vi "ook.vi"() -> ()   [LabVIEW 2009]
panel:
  out "合成波":cluster{dbl[], dbl[]}(graph)
  out "XYグラフ 3":cluster{dbl[], dbl[]}(graph) caption="XYグラフ"
  out "XYグラフ 2":cluster{dbl[], dbl[]}(graph) caption="XYグラフ"
  out "XYグラフ":cluster{dbl[], dbl[]}(graph)
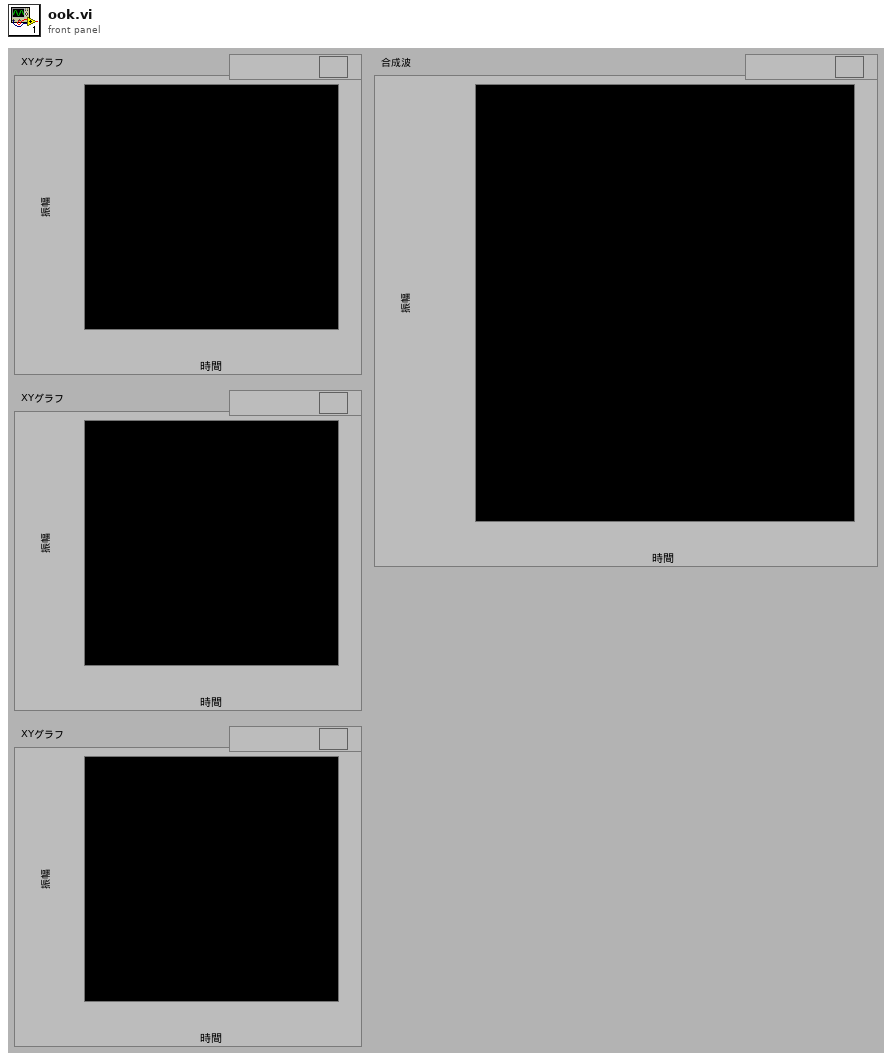
[diagram p1: front panel]
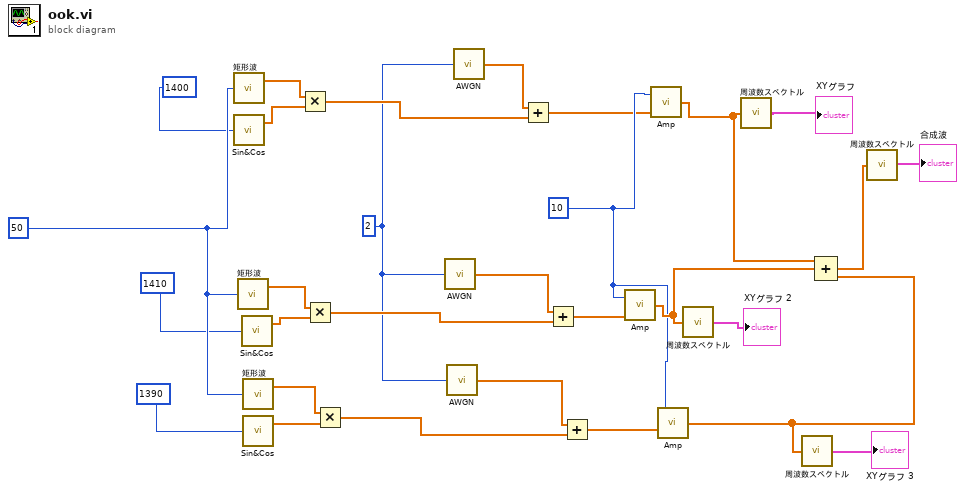
[diagram p0: block diagram]
diagram:
  w1 = 2
  w11 = 10
  w23 = 50
  n1 = call "矩形波.vi"("信号周波数 [kHz]"=w23) -> ("矩形波"=w24:dbl[])  [unwired: 1 out]
  n2 = call "Sin&Cos.vi"("周波数[kHz]"=1400) -> ("sin"=w25:dbl[])  [unwired: 1 out]
  n3 = call "矩形波.vi"("信号周波数 [kHz]"=w23) -> ("矩形波"=w27:dbl[])  [unwired: 1 out]
  n4 = call "Sin&Cos.vi"("周波数[kHz]"=1410) -> ("sin"=w26:dbl[])  [unwired: 1 out]
  n5 = call "矩形波.vi"("信号周波数 [kHz]"=w23) -> ("矩形波"=w28:dbl[])  [unwired: 1 out]
  n6 = call "Sin&Cos.vi"("周波数[kHz]"=1390) -> ("sin"=w29:dbl[])  [unwired: 1 out]
  n7 = Multiply(x=w24, y=w25) -> (x*y=w9:dbl[])
  n8 = Multiply(x=w27, y=w26) -> (x*y=w6:dbl[])
  n9 = Multiply(x=w28, y=w29) -> (x*y=w4:dbl[])
  n10 = call "AWGN.vi"("振幅値"=w1) -> ("出力"=w7:dbl[])
  n11 = call "AWGN.vi"("振幅値"=w1) -> ("出力"=w5:dbl[])
  n12 = call "AWGN.vi"("振幅値"=w1) -> ("出力"=w10:dbl[])
  n13 = Add(x=w10, y=w9) -> (x+y=w8:dbl[])
  n14 = Add(x=w7, y=w6) -> (x+y=w2:dbl[])
  n15 = Add(x=w5, y=w4) -> (x+y=w3:dbl[])
  n16 = call "Amp.vi"("入力"=w2, "増幅率"=w11) -> ("出力"=w13:dbl[])
  n17 = call "Amp.vi"("入力"=w8, "増幅率"=w11) -> ("出力"=w14:dbl[])
  n18 = call "Amp.vi"("入力"=w3, "増幅率"=w11) -> ("出力"=w12:dbl[])
  n19 = call "周波数スペクトル.vi"("入力"=w13) -> ("周波数スペクトル"=→"XYグラフ 2":cluster{dbl[], dbl[]})
  n20 = call "周波数スペクトル.vi"("入力"=w14) -> ("周波数スペクトル"=→"XYグラフ":cluster{dbl[], dbl[]})
  n21 = call "周波数スペクトル.vi"("入力"=w12) -> ("周波数スペクトル"=→"XYグラフ 3":cluster{dbl[], dbl[]})
  n22 = Compound Arithmetic op=ADD(w14, w13, w12) -> (w17:dbl[])
  n23 = call "周波数スペクトル.vi"("入力"=w17) -> ("周波数スペクトル"=→"合成波":cluster{dbl[], dbl[]})
